vi "GVAIs.vi"() -> ()   [LabVIEW 2010]
panel:
  in  "AIs":dbl[](array[numeric])
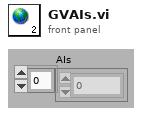
[diagram p1: front panel]
diagram:
